vi "Graph.vi"() -> ()   [LabVIEW 2019]
panel:
  in  "曲线":cluster{"X轴":dbl[], "Y轴":dbl[]}
  in  "GraphPosition":i32
  out "XY图":cluster{"X轴":dbl[], "Y轴":dbl[]}[](graph)
  in  "OK":bool
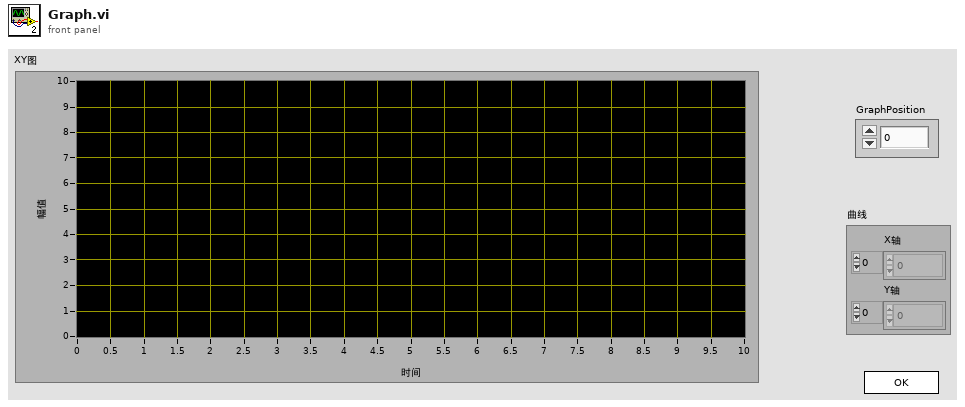
[diagram p1: front panel]
types:
  T1 = enum32{"invalid app kind", "Development System", "Run Time System", "Student Edition", "Embedded LabVIEW", "Evaluation", "Custom"}
  T2 = enum32{"Invalid", "Standard", "Closed", "Hidden", "Minimized", "Maximized"}
  T3 = cluster{"Core":cluster{"Current VI Reference":refnum<vi>, "Close Panel on Exit?":bool}, "Your Boolean data":bool, "Your string data":string}
  T4 = cluster{"Current VI Reference":refnum<vi>, "Close Panel on Exit?":bool}
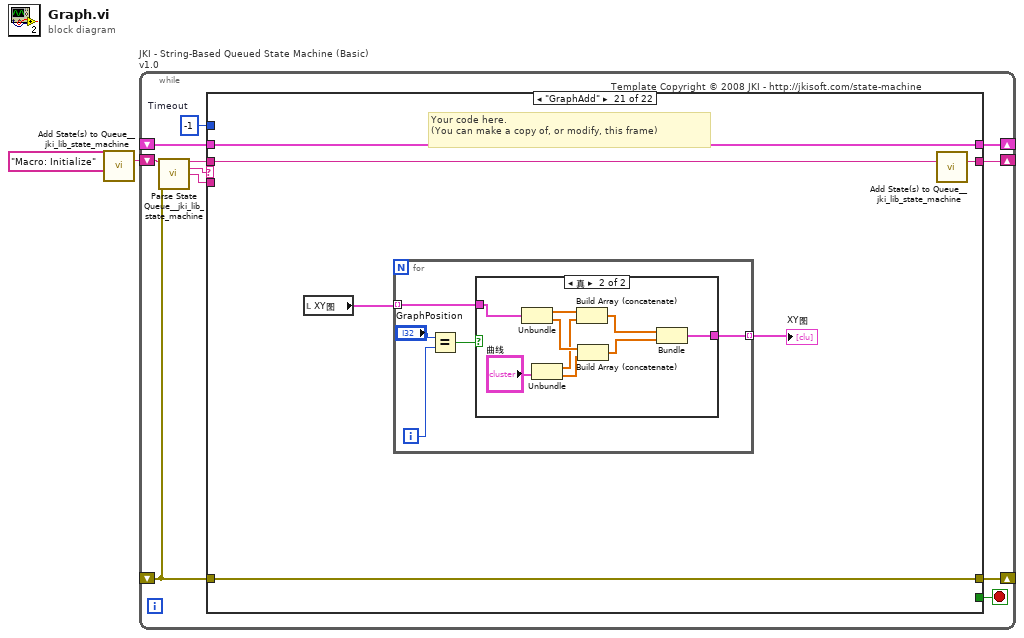
[diagram p0: block diagram]
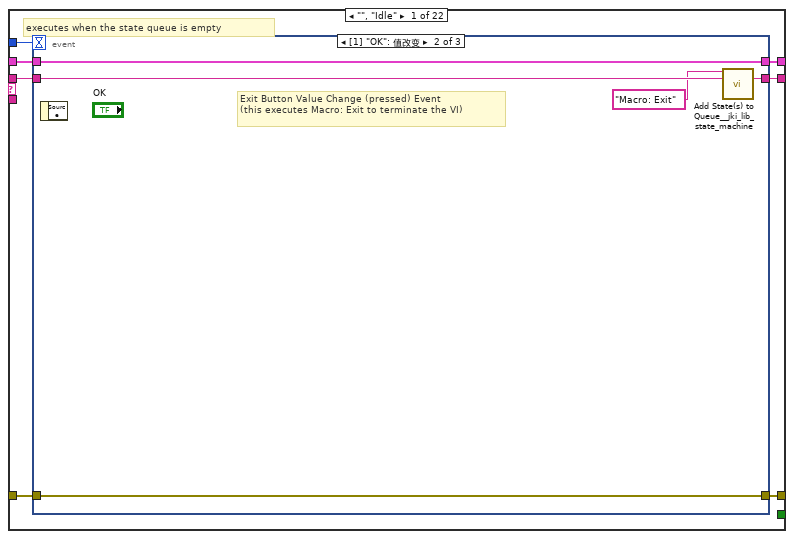
[diagram p2: hidden frame]
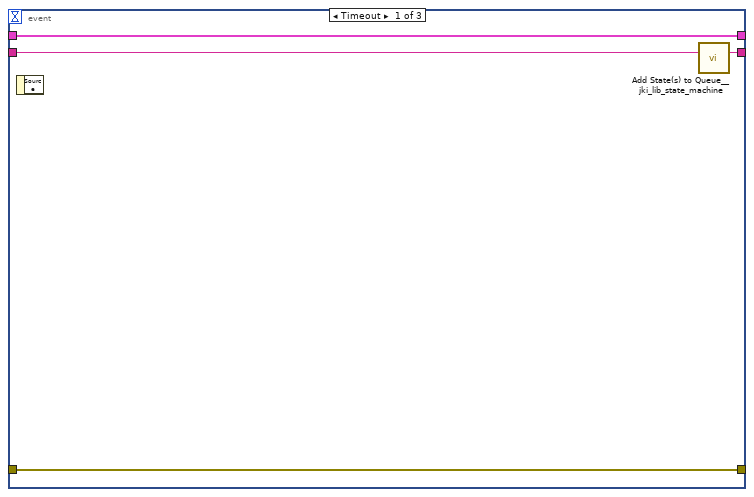
[diagram p3: hidden frame]
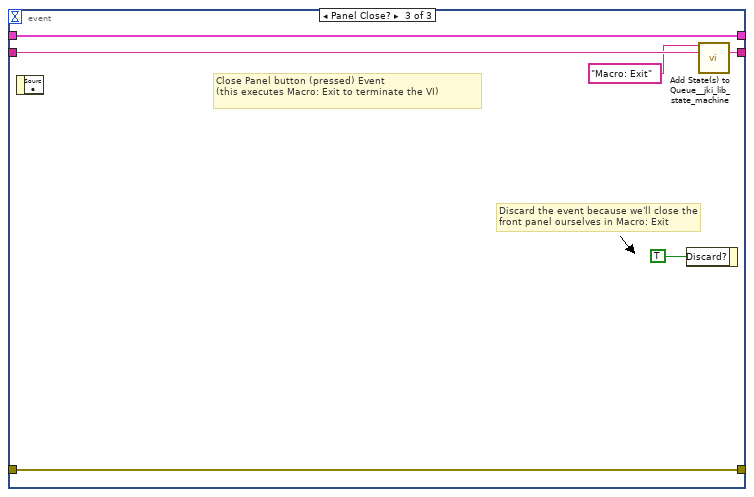
[diagram p4: hidden frame]
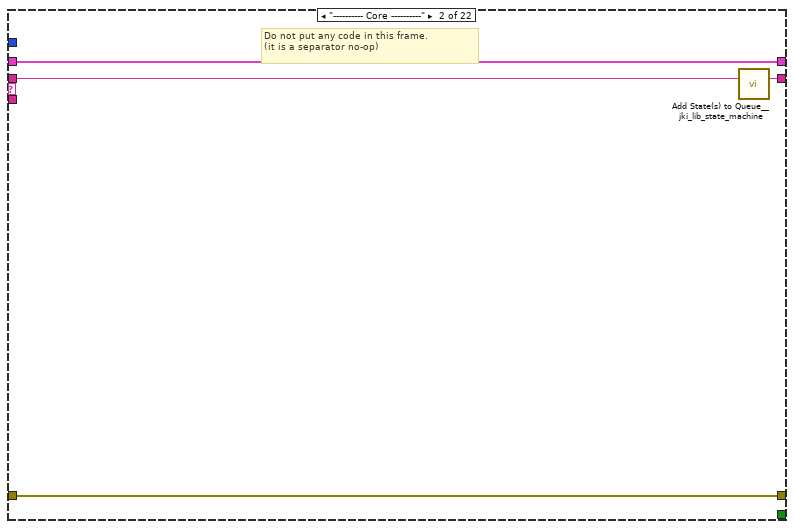
[diagram p5: hidden frame]
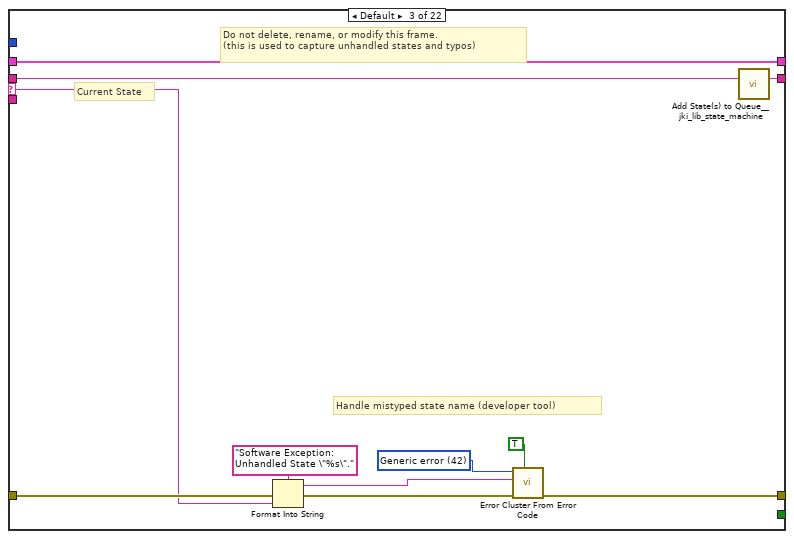
[diagram p6: hidden frame]
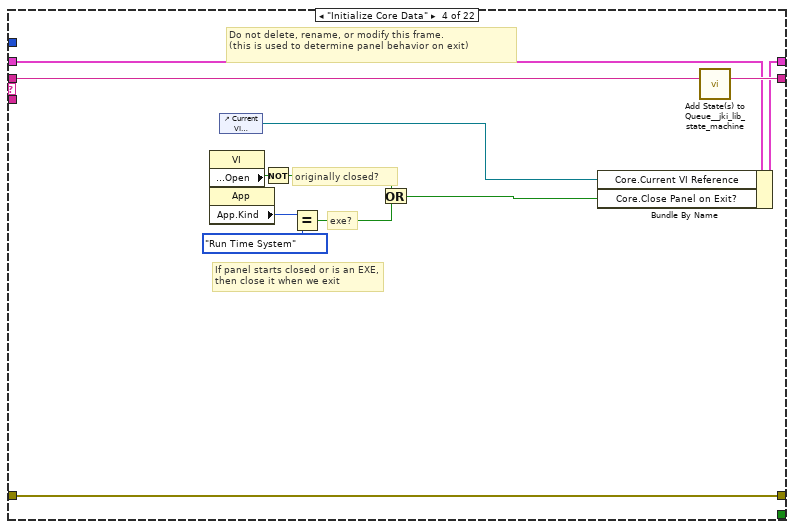
[diagram p7: hidden frame]
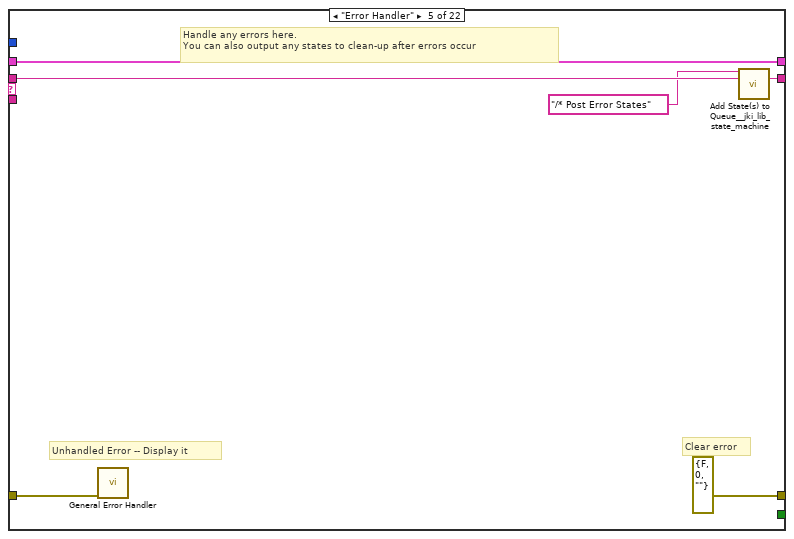
[diagram p8: hidden frame]
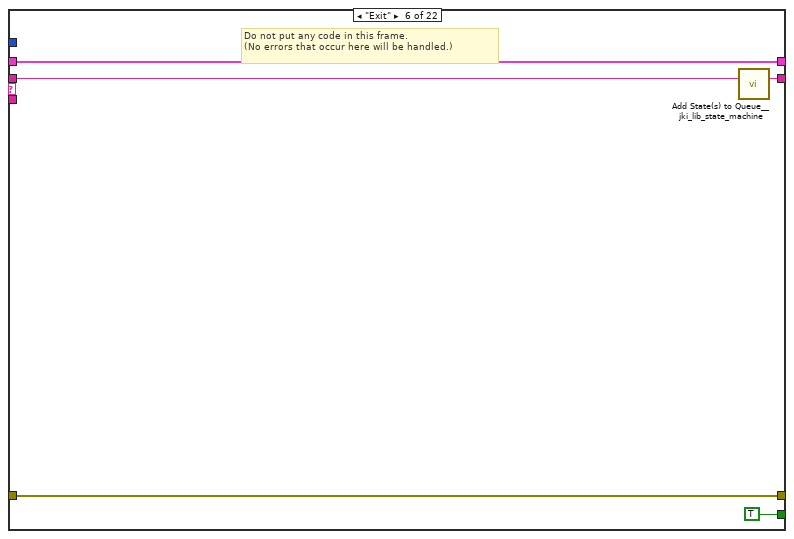
[diagram p9: hidden frame]
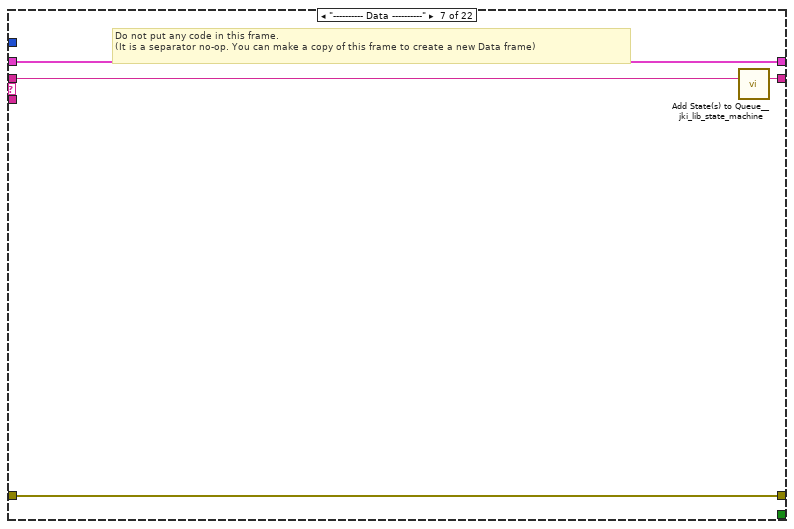
[diagram p10: hidden frame]
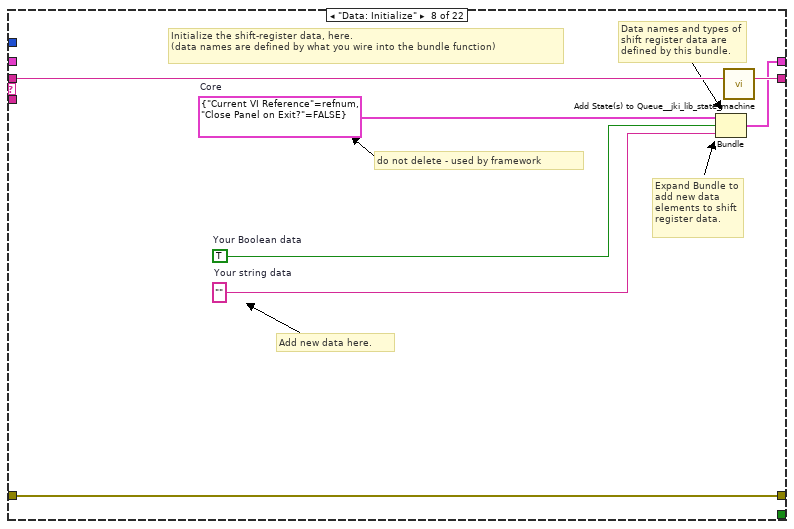
[diagram p11: hidden frame]
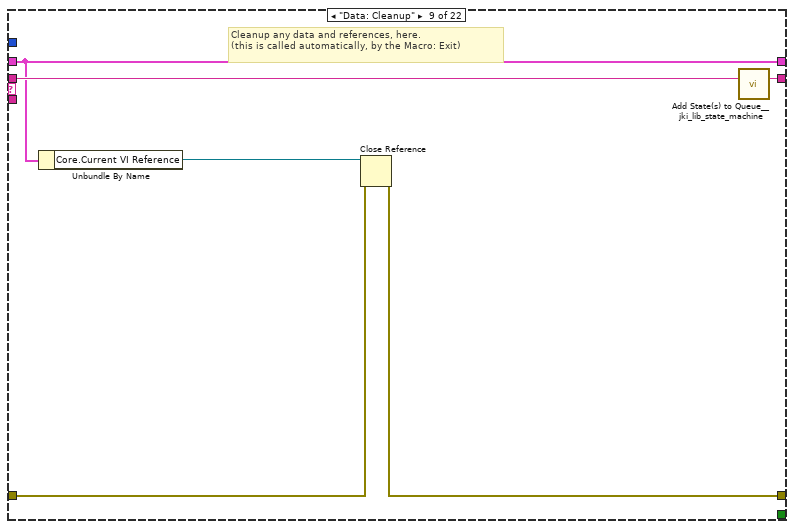
[diagram p12: hidden frame]
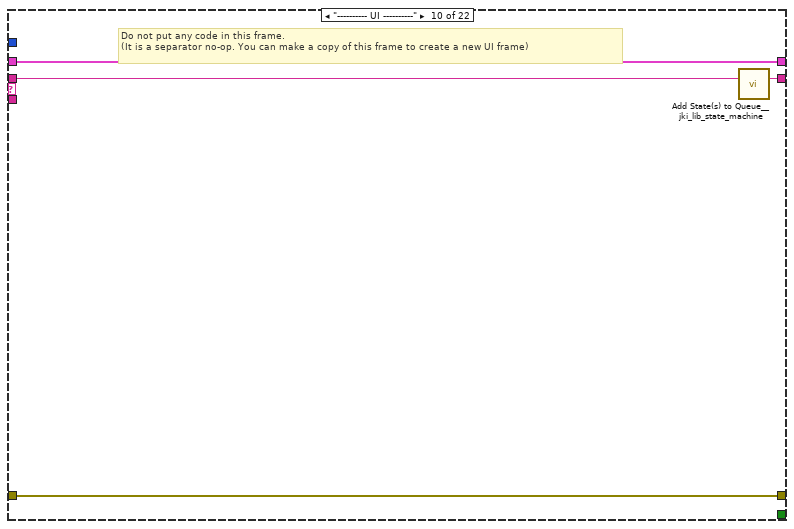
[diagram p13: hidden frame]
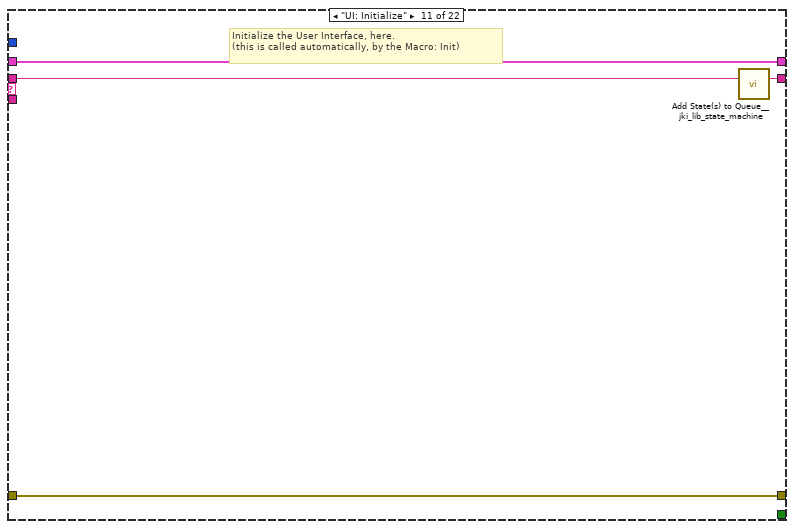
[diagram p14: hidden frame]
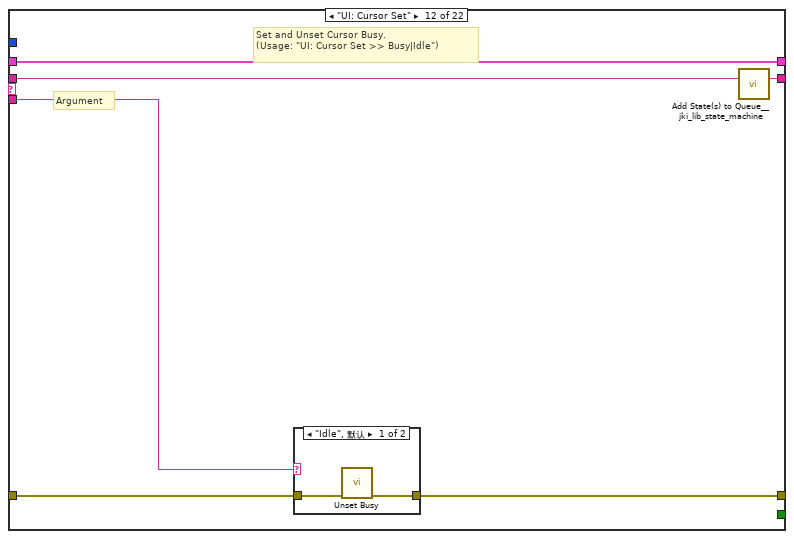
[diagram p15: hidden frame]
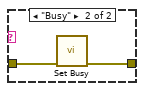
[diagram p16: hidden frame]
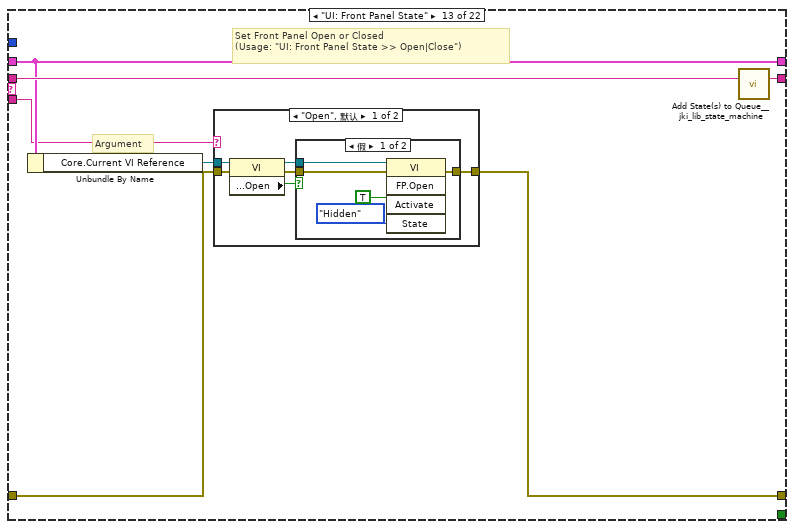
[diagram p17: hidden frame]
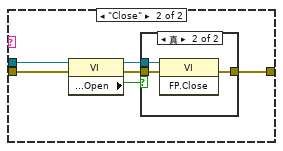
[diagram p19: hidden frame]
diagram:
  n1 = call <vilib>:"Add State(s) to Queue__jki_lib_state_machine.vi"("State(s) in (\"\")"="Macro: Initialize") -> ("States Out"=w2:string)  [unwired: 14 in]
  n2 = while "JKI - String-Based Queued State Machine (Basic) v1.0" {
    shift-right: [w6] -> _
    shift-left: _ -> [w5]
    shift-right: [w9] -> _
    shift-left: _ -> [w3]
    shift-right: [w8] -> _
    shift-left: w2 -> [w10]
    stop <- w7 stop-if-true
    w4 = -1  # Timeout
    # "Template Copyright © 2008 JKI - http://jkisoft.com/state-machine"
    n3 = call <vilib>:"Parse State Queue__jki_lib_state_machine.vi"("State Queue"=w10, "Error In (no error)"=w3) -> ("Remaining States"=w12:string, "Current State"=w13:string, "Arguments"=w11:string)  [unwired: 11 in]
    n4 = case shown="\"GraphAdd\"" w13 {
      selector: w13 -> [_ _ w40 _ _ _ _ _ _ _ _ _ _ _ _ _ _ _ _ _ _ _]
      tunnel: w12 -> [w20 w39 w44 w62 w68 w73 w77 w84 w90 w94 w98 w104 w115 w141 w146 w156 w160 w164 w168 w172 w178 w198]
      tunnel: w11 -> [_ _ _ _ _ _ _ _ _ _ _ w99 w109 _ _ _ _ _ _ _ _ _]
      tunnel: w5 -> [w18 w36 w42 w53 w65 w71 w74 _ w85 w91 w96 w102 w111 w138 w143 w153 w157 w161 w165 w169 w176 w196]
      tunnel: [w17 w37 w46 w59 errorcluster {"status"=FALSE, "code"=0, "source"=""} ("error out") w70 w75 w81 w86 w92 w95 w100 w112 w139 w144 w154 w158 w162 w166 w170 w175 w195] -> w9
      tunnel: w3 -> [w16 w37 w45 w59 w64 w70 w75 w81 w87 w92 w95 w101 w113 w139 w144 w154 w158 w162 w166 w170 w175 w195]
      tunnel: [w19 w38 w43 w61 w67 w72 w76 w83 w89 w93 w97 w103 w114 w140 w145 w155 w159 w163 w167 w171 w177 w197] -> w8
      tunnel: [_ _ _ _ _ TRUE _ _ _ _ _ _ _ _ _ _ _ _ _ _ _ _] -> w7
      tunnel: [w15 w36 w42 w60 w65 w71 w74 w82 w85 w91 w96 w102 w111 w138 w143 w153 w157 w161 w165 w169 w176 w196] -> w6
      tunnel: w4 -> [w14 _ _ _ _ _ _ _ _ _ _ _ _ _ _ _ _ _ _ _ _ _]
      frame "", "Idle" {
        # "executes when the state queue is empty"
        n5 = event shown="[1] \"OK\": 值改变" {
          selector: _ -> [_ _ _]
          dyn-events: _ -> [_ _ _]
          timeout: w14 -> [_ _ _]
          tunnel: w20 -> [w24 w29 w35]
          tunnel: [w23 w28 w34] -> w19
          tunnel: w18 -> [w21 w26 w32]
          tunnel: [w22 w27 w33] -> w17
          tunnel: w16 -> [w22 w27 w33]
          tunnel: [w21 w26 w32] -> w15
          event Timeout {
            n6 = event-data() -> ()  [unwired: 1 in, 1 out]
            n7 = call <vilib>:"Add State(s) to Queue__jki_lib_state_machine.vi"("State(s) in (\"\")"=w24) -> ("States Out"=w23:string)  [unwired: 14 in]
          }
          event "OK": Value Change {
            # "Exit Button Value Change (pressed) Event\n(this executes Macro: Exit to terminate the VI)"
            n8 = event-data() -> ()  [unwired: 1 in, 1 out]
            n9 = call <vilib>:"Add State(s) to Queue__jki_lib_state_machine.vi"("State(s) in Front (\"\")"="Macro: Exit", "State(s) in (\"\")"=w29) -> ("States Out"=w28:string)  [unwired: 13 in]
          }
          event Panel Close? {
            # "Discard the event because we'll close the front panel ourselves in Macro: Exit"
            # "Close Panel button (pressed) Event\n(this executes Macro: Exit to terminate the VI)"
            n10 = event-data() -> ()  [unwired: 1 in, 1 out]
            n11 = event-data("Discard?"=TRUE) -> ()  [unwired: 1 in, 1 out]
            n12 = call <vilib>:"Add State(s) to Queue__jki_lib_state_machine.vi"("State(s) in Front (\"\")"="Macro: Exit", "State(s) in (\"\")"=w35) -> ("States Out"=w34:string)  [unwired: 13 in]
          }
        }
      }
      frame "---------- Core ----------" {
        # "Do not put any code in this frame.\n(it is a separator no-op)"
        n13 = call <vilib>:"Add State(s) to Queue__jki_lib_state_machine.vi"("State(s) in (\"\")"=w39) -> ("States Out"=w38:string)  [unwired: 14 in]
      }
      frame Default {
        w49 = 42 items=["No error", "Argument error", "Memory is full", "Out of zone", "End of file", "File already open", "Generic file I/O error", "File not found", "File permission error", "Disk is full", "Duplicate path", "Too many files open", "System feature not enabled", "Resource file not found", "Cannot add resource", "Resource not found", "Image not found", "Image memory error", "Pen does not exist", "Config type invalid", "Config token not found", "Config parse error", "Config memory error", "Bad external code format", "Bad external code offset", "External code not present", "Null window", "Destroy window error", "Null menu", "Print aborted", "Bad print record", "Print driver error", "Windows error during printing", "Memory error during printing", "Print dialog error", "Generic print error", "Invalid device refnum", "Device not found", "Device parameter error", "Device unit error", "Cannot open device", "Device call aborted", "Generic error", "Cancelled by user", "Object ID too low", "Object ID too high", "Object not in heap", "Unknown heap", "Unknown object (invalid DefProc)", "Unknown object (DefProc not in table)", "Message out of range", "Invalid (null) method", "Unknown message", "Manager call not supported", "Bad address", "Network operation in progress", "Network operation timed out", "Connection is busy", "Network attribute not supported", "Network error", "Address in use", "System out of memory", "Connection aborted", "Connection refused", "Not connected", "Already connected", "Connection closed", "Initialization error (interapplication manager)", "Bad occurrence", "Wait on unbound occurrence handler", "Occurrence queue overflow", "Datalog type conflict", "Unused", "Unrecognized type (interapplication manager)", "Memory corrupt", "Failed to make temporary DLL", "Old CIN version", "Drag socket not found", "Failed to load drop-object", "Failed to register OLE object", "Failed to release OLE object", "Format specifier type mismatch", "Unknown format specifier", "Too few format specifiers", "Too many format specifiers", "Scan failed", "Newer CIN version", "Error converting to variant", "Runtime menu error", "Password tampered", "Variant attribute not found", "Incompatible variant data type", "Event data is not available", "Event Store is not present", "Occurrence is not found", "Event Queue is not created", "Event info is not available", "Refnum passed is NULL", "Error retrieving Class GUID", "Error retrieving CoClass GUID", "Error retrieving TypeLib GUID.", "Bad built application magic bytes.", "Specific driver is different from the specific driver associated with the Logical Name.", "There is no session opened to the class driver.", "Max Error", "MAX - Error with config objects", "MAX - Error loading configuration", "MAX - Group not supported"]
        # "Current State"
        # "Do not delete, rename, or modify this frame.\n(this is used to capture unhandled states and typos)"
        # "Handle mistyped state name (developer tool)"
        n14 = Format Into String(format string="Software Exception: Unhandled State \"%s\"." ("message"), error in=w45, w40) -> (resulting string=w48:string, error out=w47:errorcluster)  [unwired: 1 in]
        n15 = call <vilib>:"Error Cluster From Error Code.vi"("show call chain? (False)"=TRUE, "error in (no error)"=w47, "error message (\"\")"=w48, "error code (0)"=w49) -> ("error out"=w46:errorcluster)  [unwired: 5 in]
        n16 = call <vilib>:"Add State(s) to Queue__jki_lib_state_machine.vi"("State(s) in (\"\")"=w44) -> ("States Out"=w43:string)  [unwired: 14 in]
      }
      frame "Initialize Core Data" {
        # "Do not delete, rename, or modify this frame.\n(this is used to determine panel behavior on exit)"
        # "originally closed?"
        # "exe?"
        # "If panel starts closed or is an EXE, then close it when we exit"
        n17 = property class="VI"() -> ("Front Panel.Open"=w58:bool)  [unwired: 2 in, 2 out]
        n18 = property class="App"() -> ("App.Kind"=w57:T1)  [unwired: 2 in, 2 out]
        n19 = control-ref of="Current VI Reference"() -> (w51:refnum<vi>)
        n20 = Not(x=w58) -> (.not. x?=w55:bool)
        n21 = Equal?(x=w57, y=T1."Run Time System" ("Application:Kind")) -> (x = y?=w54:bool)
        n22 = Or(x=w55, y=w54) -> (x .or. y?=w52:bool)
        n23 = Bundle By Name(cluster=w53, "Core.Current VI Reference"=w51, "Core.Close Panel on Exit?"=w52) -> (w60:T3)
        n24 = call <vilib>:"Add State(s) to Queue__jki_lib_state_machine.vi"("State(s) in (\"\")"=w62) -> ("States Out"=w61:string)  [unwired: 14 in]
      }
      frame "Error Handler" {
        # "Unhandled Error -- Display it"
        # "Handle any errors here.\nYou can also output any states to clean-up after errors occur"
        # "Clear error"
        n25 = call <vilib>:"General Error Handler.vi"("error in (no error)"=w64) -> ()  [unwired: 10 in, 5 out]
        n26 = call <vilib>:"Add State(s) to Queue__jki_lib_state_machine.vi"("State(s) in Front (\"\")"="/* Post Error States", "State(s) in (\"\")"=w68) -> ("States Out"=w67:string)  [unwired: 13 in]
      }
      frame "Exit" {
        # "Do not put any code in this frame.\n(No errors that occur here will be handled.)"
        n27 = call <vilib>:"Add State(s) to Queue__jki_lib_state_machine.vi"("State(s) in (\"\")"=w73) -> ("States Out"=w72:string)  [unwired: 14 in]
      }
      frame "---------- Data ----------" {
        # "Do not put any code in this frame.\n(It is a separator no-op. You can make a copy of this frame to create a new Data frame)"
        n28 = call <vilib>:"Add State(s) to Queue__jki_lib_state_machine.vi"("State(s) in (\"\")"=w77) -> ("States Out"=w76:string)  [unwired: 14 in]
      }
      frame "Data: Initialize" {
        w78 = T4 {"Current VI Reference"=refnum, "Close Panel on Exit?"=FALSE}  # Core
        w80 = TRUE  # Your Boolean data
        w79 = ""  # Your string data
        # "do not delete - used by framework"
        # "Expand Bundle to add new data elements to shift register data."
        # "Add new data here."
        # "Data names and types of shift register data are defined by this bundle."
        # "Initialize the shift-register data, here.\n(data names are defined by what you wire into the bundle function)"
        n29 = Bundle("Core"=w78, "Your Boolean data"=w80, "Your string data"=w79) -> (w82:T3)  [unwired: 1 in]
        n30 = call <vilib>:"Add State(s) to Queue__jki_lib_state_machine.vi"("State(s) in (\"\")"=w84) -> ("States Out"=w83:string)  [unwired: 14 in]
      }
      frame "Data: Cleanup" {
        # "Cleanup any data and references, here.\n(this is called automatically, by the Macro: Exit)"
        n31 = Unbundle By Name(w85) -> ("Core.Current VI Reference"=w88:refnum<vi>)
        n32 = Close Reference(reference=w88, error in (no error)=w87) -> (error out=w86:errorcluster)
        n33 = call <vilib>:"Add State(s) to Queue__jki_lib_state_machine.vi"("State(s) in (\"\")"=w90) -> ("States Out"=w89:string)  [unwired: 14 in]
      }
      frame "---------- UI ----------" {
        # "Do not put any code in this frame.\n(It is a separator no-op. You can make a copy of this frame to create a new UI frame)"
        n34 = call <vilib>:"Add State(s) to Queue__jki_lib_state_machine.vi"("State(s) in (\"\")"=w94) -> ("States Out"=w93:string)  [unwired: 14 in]
      }
      frame "UI: Initialize" {
        # "Initialize the User Interface, here.\n(this is called automatically, by the Macro: Init)"
        n35 = call <vilib>:"Add State(s) to Queue__jki_lib_state_machine.vi"("State(s) in (\"\")"=w98) -> ("States Out"=w97:string)  [unwired: 14 in]
      }
      frame "UI: Cursor Set" {
        # "Argument"
        # "Set and Unset Cursor Busy.\n(Usage: \"UI: Cursor Set >> Busy|Idle\")"
        n36 = case shown="\"Idle\", 默认" w99 {
          tunnel: w101 -> [w106 w108]
          tunnel: [w105 w107] -> w100
          frame "Idle", Default {
            n37 = call <vilib>:"Unset Busy.vi"("error in (no error)"=w106) -> ("error out"=w105:errorcluster)  [unwired: 10 in]
          }
          frame "Busy" {
            n38 = call <vilib>:"Set Busy.vi"("error in (no error)"=w108) -> ("error out"=w107:errorcluster)  [unwired: 9 in, 1 out]
          }
        }
        n39 = call <vilib>:"Add State(s) to Queue__jki_lib_state_machine.vi"("State(s) in (\"\")"=w104) -> ("States Out"=w103:string)  [unwired: 14 in]
      }
      frame "UI: Front Panel State" {
        # "Argument"
        # "Set Front Panel Open or Closed\n(Usage: \"UI: Front Panel State >> Open|Close\")"
        n40 = Unbundle By Name(w111) -> ("Core.Current VI Reference"=w110:refnum<vi>)
        n41 = case shown="\"Open\", 默认" w109 {
          tunnel: w113 -> [w119 w132]
          tunnel: [w121 w133] -> w112
          tunnel: w110 -> [w120 w130]
          frame "Open", Default {
            n42 = property class="VI"(reference=w120, error in=w119) -> (reference out=w117:refnum<vi>, error out=w118:errorcluster, "Front Panel.Open"=w116:bool)
            n43 = case shown="假" w116 {
              tunnel: [w124 w127] -> w121
              tunnel: w118 -> [w123 w127]
              tunnel: w117 -> [w122 _]
              frame False {
                n44 = invoke class="VI" method="FP.Open"(reference=w122, error in=w123, "Activate"=TRUE, "State"=T2."Hidden") -> (error out=w124:errorcluster)  [unwired: 1 in, 4 out]
              }
              frame True {
              }
            }
          }
          frame "Close" {
            n45 = property class="VI"(reference=w130, error in=w132) -> (reference out=w129:refnum<vi>, error out=w131:errorcluster, "Front Panel.Open"=w128:bool)
            n46 = case shown="真" w128 {
              tunnel: [w134 w137] -> w133
              tunnel: w131 -> [w134 w136]
              tunnel: w129 -> [_ w135]
              frame False {
              }
              frame True {
                n47 = invoke class="VI" method="FP.Close"(reference=w135, error in=w136) -> (error out=w137:errorcluster)  [unwired: 1 in, 2 out]
              }
            }
          }
        }
        n48 = call <vilib>:"Add State(s) to Queue__jki_lib_state_machine.vi"("State(s) in (\"\")"=w115) -> ("States Out"=w114:string)  [unwired: 14 in]
      }
      frame "---------- Macro ----------" {
        # "Do not put any code in this frame.\n(It is a separator no-op. You can make a copy of this frame to create a new Macro frame)"
        n49 = call <vilib>:"Add State(s) to Queue__jki_lib_state_machine.vi"("State(s) in (\"\")"=w141) -> ("States Out"=w140:string)  [unwired: 14 in]
      }
      frame "Macro: Initialize" {
        w142 = "Data: Initialize\nInitialize Core Data\nUI: Initialize\nUI: Front Panel State >> Open"  # Data: Initialize Initialize Core Data UI: Initialize UI: Front Panel State >> Open
        # "Initialization Macro\n(This is called once, when the VI starts)"
        n50 = call <vilib>:"Add State(s) to Queue__jki_lib_state_machine.vi"("State(s) in Front (\"\")"=w142, "State(s) in (\"\")"=w146) -> ("States Out"=w145:string)  [unwired: 13 in]
      }
      frame "Macro: Exit" {
        # "Exit Macro\n(This is called once, when the VI exits)"
        n51 = Unbundle By Name(w153) -> ("Core.Close Panel on Exit?"=w152:bool)
        n52 = Select(t="UI: Front Panel State >> Close", s=w152, f="") -> (s? t:f=w149:string)
        n53 = call <vilib>:"Add State(s) to Queue__jki_lib_state_machine.vi"("State(s) in (\"\")"=w149, "State(s) at Back (\"\")"="Data: Cleanup\nExit") -> ("States Out"=w147:string)  [unwired: 13 in]
        n54 = call <vilib>:"Add State(s) to Queue__jki_lib_state_machine.vi"("State(s) in Front (\"\")"=w147, "State(s) in (\"\")"=w156) -> ("States Out"=w155:string)  [unwired: 13 in]
      }
      frame "---------- New Category ----------" {
        # "Template Separator\n(You can make a copy of, or modify, this frame)"
        n55 = call <vilib>:"Add State(s) to Queue__jki_lib_state_machine.vi"("State(s) in (\"\")"=w160) -> ("States Out"=w159:string)  [unwired: 14 in]
      }
      frame "New Category: 1" {
        # "Your code here.\n(You can make a copy of, or modify, this frame)"
        n56 = call <vilib>:"Add State(s) to Queue__jki_lib_state_machine.vi"("State(s) in (\"\")"=w164) -> ("States Out"=w163:string)  [unwired: 14 in]
      }
      frame "New Category: 2" {
        # "Your code here.\n(You can make a copy of, or modify, this frame)"
        n57 = call <vilib>:"Add State(s) to Queue__jki_lib_state_machine.vi"("State(s) in (\"\")"=w168) -> ("States Out"=w167:string)  [unwired: 14 in]
      }
      frame "--------Graph---------" {
        # "Template Separator\n(You can make a copy of, or modify, this frame)"
        n58 = call <vilib>:"Add State(s) to Queue__jki_lib_state_machine.vi"("State(s) in (\"\")"=w172) -> ("States Out"=w171:string)  [unwired: 14 in]
      }
      frame "GraphAdd" {
        # "Your code here.\n(You can make a copy of, or modify, this frame)"
        n59 = local read "XY图"() -> (w174:cluster{"X轴":dbl[], "Y轴":dbl[]}[])
        n60 = for {
          tunnel: w174 -> [w183] mode=indexing
          tunnel: [w182] -> w173 mode=indexing
          i -> [w180]
          n61 = Equal?(x="GraphPosition", y=w180) -> (x = y?=w181:bool)
          n62 = case shown="真" w181 {
            tunnel: w183 -> [w184 w191]
            tunnel: [w184 w188] -> w182
            frame False {
            }
            frame True {
              n63 = Unbundle(w191) -> ("X轴"=w193:dbl[], "Y轴"=w192:dbl[])
              n64 = Unbundle("曲线") -> ("X轴"=w186:dbl[], "Y轴"=w185:dbl[])
              n65 = Build Array (concatenate)(w193, w186) -> (w190:dbl[])
              n66 = Build Array (concatenate)(w192, w185) -> (w189:dbl[])
              n67 = Bundle(w190, w189) -> (w188:cluster{dbl[], dbl[]})  [unwired: 1 in]
            }
          }
        }
        "XY图" <- w173
        n68 = call <vilib>:"Add State(s) to Queue__jki_lib_state_machine.vi"("State(s) in (\"\")"=w178) -> ("States Out"=w177:string)  [unwired: 14 in]
      }
      frame "GraphClean" {
        # "Your code here.\n(You can make a copy of, or modify, this frame)"
        n69 = local write "XY图"(cluster{"X轴":dbl[], "Y轴":dbl[]}[] [] ("XY图")) -> ()
        n70 = call <vilib>:"Add State(s) to Queue__jki_lib_state_machine.vi"("State(s) in (\"\")"=w198) -> ("States Out"=w197:string)  [unwired: 14 in]
      }
    }
  }
